vi "Add_CP.vi"(6 "dl":i32=1, 8 "Sdl":i32=8, 9 "Tdl":i32=72, 10 "Ldl":i32=64, 11 "din":cdb[](array[numeric])) -> (2 "dout":cdb[](array[numeric]))   [LabVIEW 2010]
uses:
  <vilib>/imath/engines/lvmath2/RunTimeEngine/ErrorHandling/NIMS_Finalize Error.vi
  <vilib>/imath/engines/lvmath2/RunTimeEngine/BuiltInFunctions/zeros/NIMS_V=zeros(I32,I32).vi
  <vilib>/imathl/engines/lvmath/Functions/Error Handling/Create Error.vi
  <vilib>/imath/engines/lvmath2/RunTimeEngine/RangeToken/NIMS_Range_R2 - Integer.vi
  <instcachedir>/0/NIMS_Range_R2 - Integer_217CA55F27D14E80B3D190635C7B3F47.lvgen/NIMS_Range_R2 - Integer_217CA55F27D14E80B3D190635C7B3F47_000.vi
  <vilib>/imath/engines/lvmath2/RunTimeEngine/NodeEndStatement/NIMS_NodeEndStatement_Output.vi
  <instcachedir>/0/NIMS_NodeEndStatement_Output_53EC0D466D134D7ABD903AC30B43404B.lvgen/NIMS_NodeEndStatement_Output_53EC0D466D134D7ABD903AC30B43404B_000.vi
  <vilib>/imath/engines/lvmath2/RunTimeEngine/CommandStatement/MC_CommandStatement_break.vi
  <vilib>/imath/engines/lvmath2/RunTimeEngine/RangeToken/NIMS_Range_R2.vi
  <vilib>/imath/engines/lvmath2/RunTimeEngine/ReplaceToken/NIMS_Replace - Check Linear.vi
  <instcachedir>/0/NIMS_Replace - Check Linear_662D5651E4E34E0584DA82A256193A4C.lvgen/NIMS_Replace - Check Linear_662D5651E4E34E0584DA82A256193A4C_000.vi
  <vilib>/imath/engines/lvmath2/RunTimeEngine/VariableToken/Read/NIMS_Get Elements - RV(_) - Check.vi
  <instcachedir>/0/NIMS_Get Elements - RV(_) - Check_1F6F8656162345078B1D4DC9877DFAE9.lvgen/NIMS_Get Elements - RV(_) - Check_1F6F8656162345078B1D4DC9877DFAE9_002.vi
  <vilib>/imath/engines/lvmath2/RunTimeEngine/ReplaceToken/NIMS_Replace - Size Check _(_)=VorM.vi
  <instcachedir>/0/NIMS_Replace - Size Check _(_)=VorM_4228B35EE910471DB74F3866D9D09B95.lvgen/NIMS_Replace - Size Check _(_)=VorM_4228B35EE910471DB74F3866D9D09B95_007.vi
  <vilib>/imath/engines/lvmath2/RunTimeEngine/ReplaceToken/NIMS_Replace - Assignment Check _(_)=VorM.vi
  <instcachedir>/0/NIMS_Replace - Assignment Check _(_)=VorM_C130F3B8B64B4DD7B9359A2D3A035D18.lvgen/NIMS_Replace - Assignment Check _(_)=VorM_C130F3B8B64B4DD7B9359A2D3A035D18_007.vi
  <vilib>/imath/engines/lvmath2/RunTimeEngine/ErrorHandling/NIMS_Create Error From Enums.vi
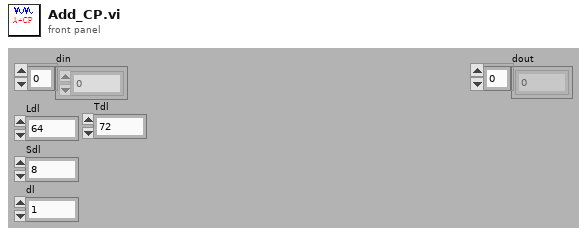
[diagram p1: front panel]
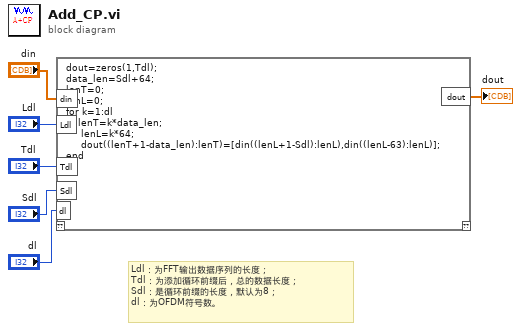
[diagram p0: block diagram]
diagram:
  # "Ldl：为FFT输出数据序列的长度；\nTdl：为添加循环前缀后，总的数据长度；\nSdl：是循环前缀的长度，默认为8；\ndl：为OFDM符号数。"
  n1 = mathscript code="dout=zeros(1,Tdl);\ndata_len=Sdl+64;\nlenT=0;\nlenL=0;\nfor k=1:dl\n    lenT=k*data_len;\n     lenL=k*64;\n     dout((lenT+1-data_len):lenT)=[din((lenL+1-Sdl):lenL),din((lenL-63):lenL)];\nend"("din"="din", "Ldl"="Ldl", "Tdl"="Tdl", "Sdl"="Sdl", "dl"="dl") -> ("dout"=→"dout":cdb[])  [unwired: 1 in, 1 out]
